vi "Report Temperature and Humidity.vi"(8 "error in (no error)":errorcluster, 9 "Humidity":dbl, 10 "Temperature":dbl, 11 "Device Manager in":refnum<class "Device Manager.lvclass">) -> (0 "error out":errorcluster, 3 "Device Manager out":refnum<class "Device Manager.lvclass">)   [LabVIEW 2020, in "Device Manager.lvlib" / "Device Manager.lvclass"]
uses:
  Device Manager.lvclass
  Device Manager.lvclass/Device Manager.ctl
  Panel/Panel Messages/Report Temperature and Humidity Msg/Report Temperature and Humidity Msg.lvclass
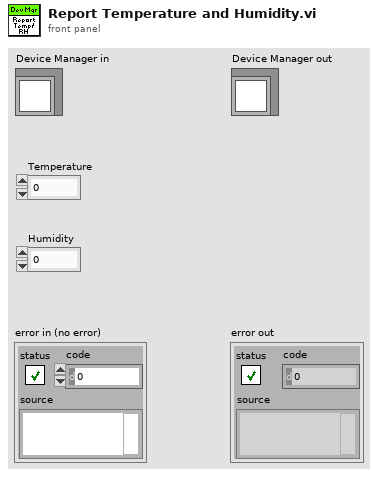
[diagram p1: front panel]
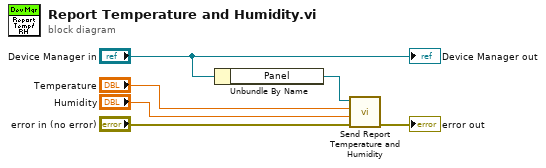
[diagram p0: block diagram]
diagram:
  n1 = Unbundle By Name("Device Manager in") -> ("Panel"=w5:refnum<class "Message Enqueuer.lvclass">)
  n2 = call "Send Report Temperature and Humidity.vi"("error in (no error)"="error in (no error)", "Humidity"="Humidity", "Temperature"="Temperature", "Message Enqueuer"=w5) -> ("error out"=→"error out":errorcluster)  [unwired: 6 in, 1 out]
  "Device Manager out" <- "Device Manager in"
